vi "Actor Core.vi"(8 "error in":errorcluster, 11 "LSR Instrument in":refnum<class "LSR Instrument.lvclass">) -> (0 "error out":errorcluster, 3 "Actor out":refnum<class "Actor.lvclass">)   [LabVIEW 2015, in "LSR Instrument.lvlib" / "LSR Instrument.lvclass"]
doc: "(<B>Filename</B>: Actor Framework.lvlib:Actor.lvclass:Actor Core.vi)\n\nReceives messages to the actor, reacts to them, and initiates any error handling that may shut the actor down.\n\nDescendant classes may override this VI to append parallel tasks for the actor to complete while it handles messages. Overrides use the Call Parent Method node."
uses:
  LSR Instrument.lvclass
  <vilib>/ActorFramework/Actor/Actor.lvclass
  LSR Instrument Messages/Send State Message Over LSR Msg/Send State Message Over LSR Msg.lvclass
  Actors/RDS Serial Instrument Actor/RDS Serial Instrument Actor.lvclass
panel:
  in  "LSR Update Time (ms)":i32=250
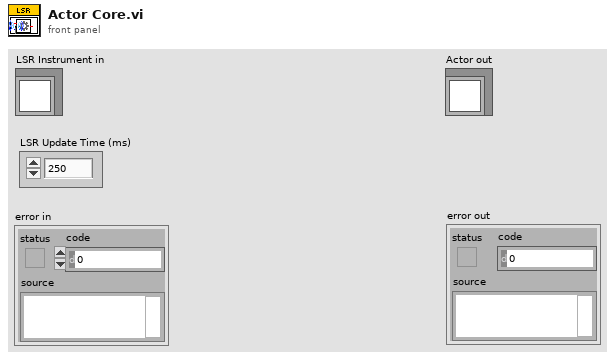
[diagram p1: front panel]
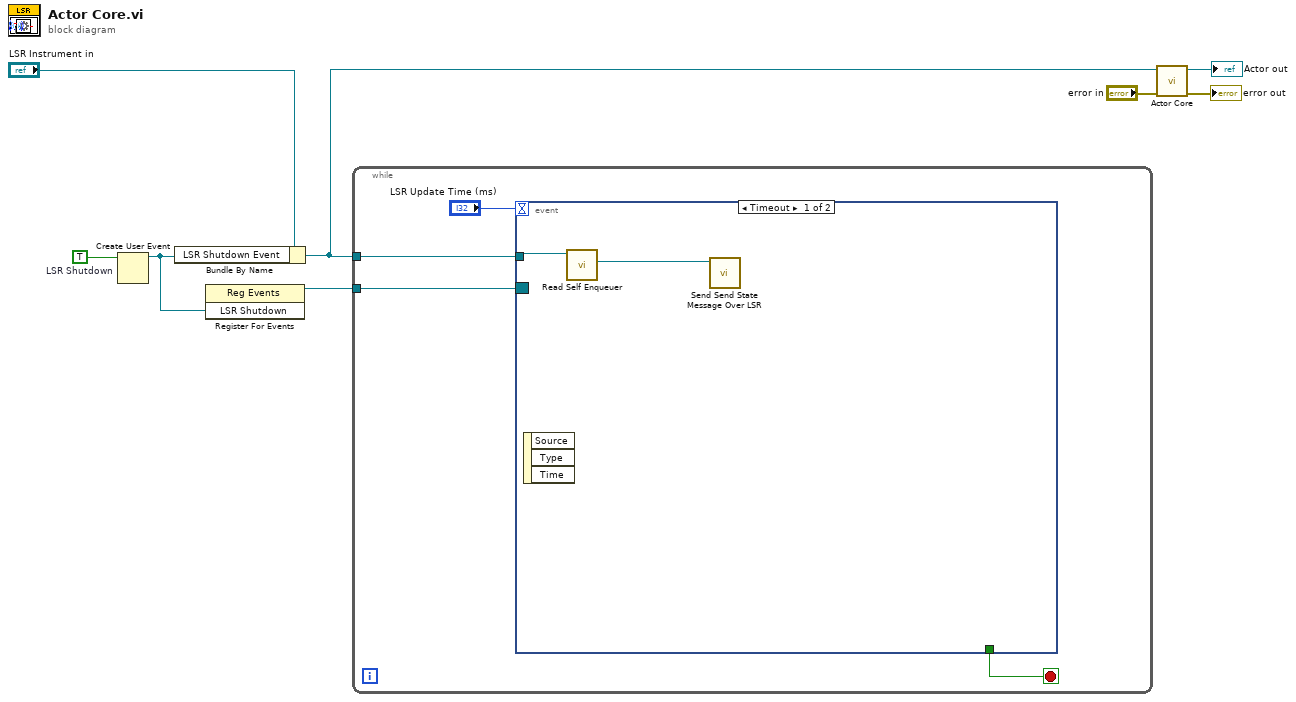
[diagram p0: block diagram]
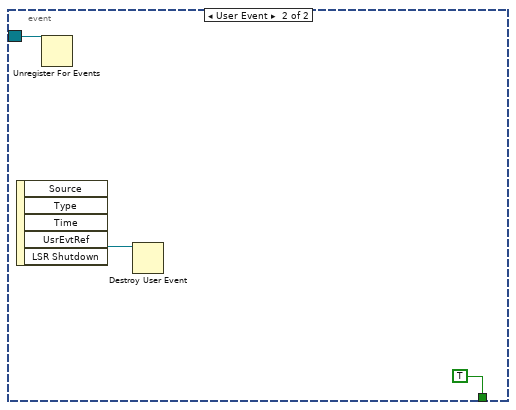
[diagram p2: hidden frame]
diagram:
  w5 = TRUE  # LSR Shutdown
  n1 = Create User Event(user event datatype=w5) -> (user event=w2:refnum<user-event>)  [unwired: 1 in, 1 out]
  n2 = Bundle By Name(cluster="LSR Instrument in", "LSR Shutdown Event"=w2) -> (w1:refnum<class "LSR Instrument.lvclass">)
  n3 = register-events(w2) -> (reference out=w3:refnum<event-registration>)  [unwired: 2 in, 1 out]
  n4 = while {
    tunnel: w3 -> [w12]
    tunnel: w1 -> [w9]
    stop <- w10 stop-if-true
    n5 = event shown="[0] Timeout" {
      selector: w12 -> [_ w16]
      dyn-events: _ -> [_ _]
      timeout: "LSR Update Time (ms)" -> [_ _]
      tunnel: [_ TRUE] -> w10
      tunnel: w9 -> [w14 _]
      event Timeout {
        n6 = event-data() -> ()  [unwired: 1 in, 3 out]
        n7 = call <vilib>:"Read Self Enqueuer.vi"("Actor"=w14) -> ("Self Enqueuer"=w13:refnum<class "Message Enqueuer.lvclass">)  [unwired: 10 in]
        n8 = call "Send Send State Message Over LSR.vi"("Message Enqueuer in"=w13) -> ()  [unwired: 9 in, 2 out]
      }
      event User Event {
        n9 = event-data() -> ("UsrEvtRef"=w15:refnum<user-event>)  [unwired: 1 in, 4 out]
        n10 = Unregister For Events(event registration refnum=w16) -> ()  [unwired: 1 in, 1 out]
        n11 = Destroy User Event(user event=w15) -> ()  [unwired: 1 in, 1 out]
      }
    }
  }
  n12 = call-parent "Actor Core.vi"("error in"="error in", "RDS Serial Instrument Actor in"=w1) -> ("error out"=→"error out":errorcluster, "Actor out"=→"Actor out":refnum<class "Actor.lvclass">)  [unwired: 8 in]
